vi "Panel Diagram.vi"() -> ()   [LabVIEW 2025]
panel:
  in  "Thermometer(DegC)":dbl(slide) scale=0.0..100.0
  in  "Stop":bool
  out "Degree Celcius(°C)":dbl
  out "Kelvin(K)":dbl
  out "Fahrenhit(F)":dbl
  out "Temperature to \nVoltage(V)":dbl
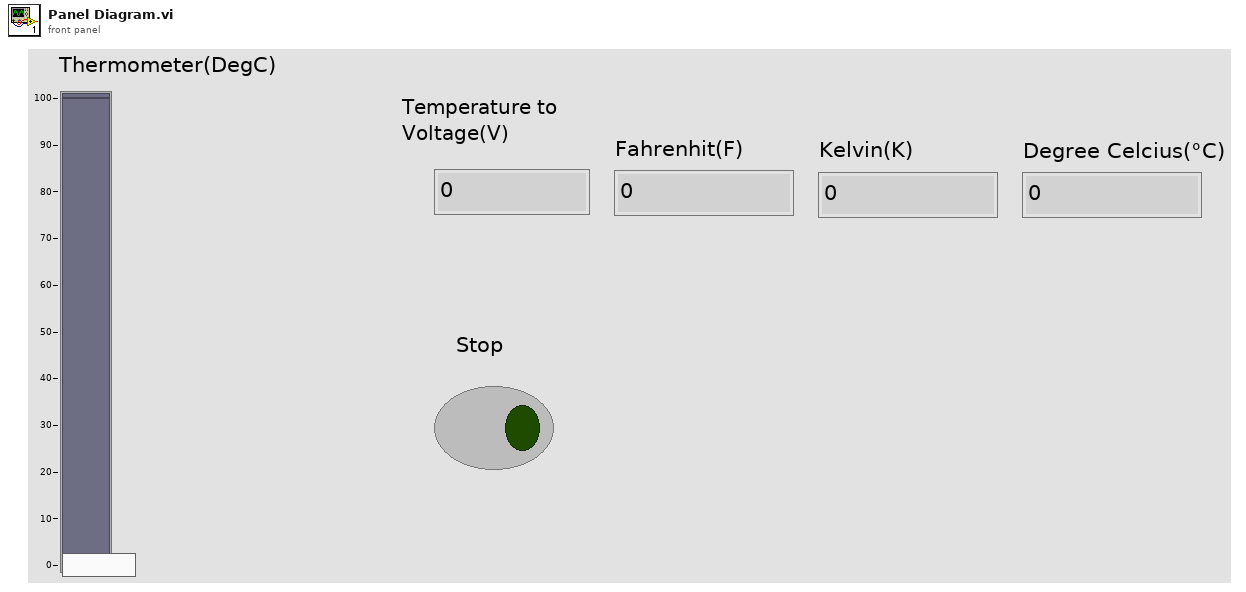
[diagram p1: front panel]
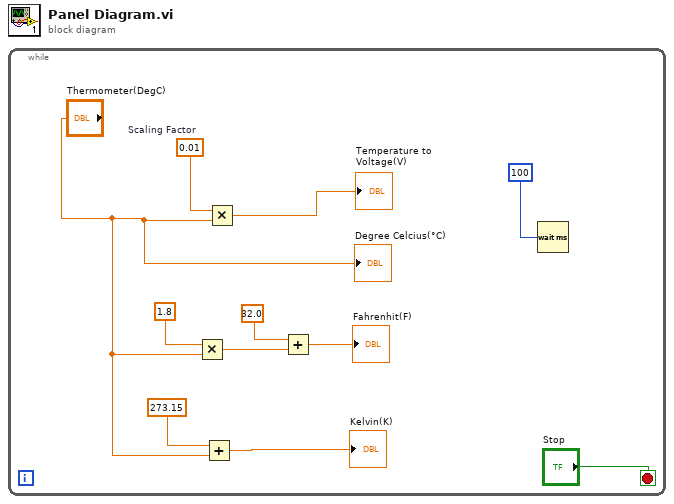
[diagram p0: block diagram]
diagram:
  n1 = while {
    stop <- "Stop" stop-if-true
    w11 = 0.01  # Scaling Factor
    n2 = Multiply(x=1.8, y="Thermometer(DegC)") -> (x*y=w9:dbl)
    n3 = Add(x=273.15, y="Thermometer(DegC)") -> (x+y=→"Kelvin(K)":dbl)
    n4 = Multiply(x=w11, y="Thermometer(DegC)") -> (x*y=→"Temperature to \nVoltage(V)":dbl)
    n5 = Add(x=32.0, y=w9) -> (x+y=→"Fahrenhit(F)":dbl)
    n6 = Wait (ms)(milliseconds to wait=u32 100) -> ()  [unwired: 1 out]
    "Degree Celcius(°C)" <- "Thermometer(DegC)"
  }
